vi "Get_T_100x.vi"(0 "error in":errorcluster) -> (2 "error out":errorcluster, 3 "Temperature Error":dbl, 4 "Temperature Mean":dbl)   [LabVIEW 2010]
uses:
  <vilib>/Analysis/NI_AALBase.lvlib
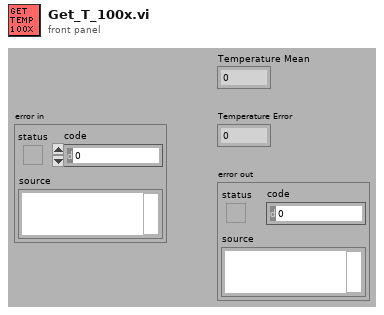
[diagram p1: front panel]
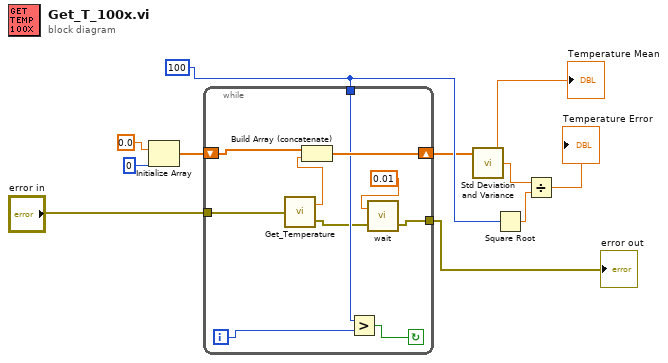
[diagram p0: block diagram]
diagram:
  w10 = 100
  n1 = Initialize Array(0.0, 0) -> (w7:dbl[])
  n2 = while {
    shift-right: [w21] -> w6
    shift-left: w7 -> [w20]
    tunnel: "error in" -> [w18]
    tunnel: w10 -> [w16]
    tunnel: [w13] -> w11
    i -> [w17]
    stop <- w15 continue-if-true
    n3 = call "Get_Temperature.vi"("error in"=w18) -> ("error out"=w14:errorcluster, "Temperature"=w19:dbl)
    n4 = Build Array (concatenate)(w20, w19) -> (w21:dbl[])
    n5 = Greater?(x=w16, y=w17) -> (0:w15:bool)
    n6 = call "wait.vi"("error in"=w14, "Wartezeit in Sek"=0.01) -> ("error out"=w13:errorcluster)  [unwired: 1 in]
  }
  "error out" <- w11
  n7 = call <vilib>:"Std Deviation and Variance.vi"("X"=w6) -> ("mean"=→"Temperature Mean":dbl, "standard deviation"=w4:dbl)  [unwired: 1 in, 1 out]
  n8 = Square Root(x=w10) -> (sqrt(x)=w3:dbl)
  n9 = Divide(x=w4, y=w3) -> (x/y=→"Temperature Error":dbl)
